vi "JKISM++ List Modules.vi"(8 "Error in":errorcluster caption="Error in (no error)", 9 "Exclude Standalone JKISM(T)":bool=TRUE) -> (0 "Error out":errorcluster, 3 "Module Names":string[](array[string]))   [LabVIEW 2014, in "JKI State Machine++.lvlib"]
doc: "List all JKISM++ Modules alive in system.\n\n<b>Inputs:</b>\n - <b>Exclude Standalone JKISM(T)</b>: 'TRUE' to exclude standalone JKISM module, and 'FALSE' to include them.\n - <b>Error in</b>: Error cluster\n\n<b>Outputs:</b>\n - <b>Module Names</b>: Module Names\n - <b>Error out</b>: Error cluster"
uses:
  JKI State Machine++.lvlib
  _Support/JKISMQ/_JKISMQFGVOPER.ctl
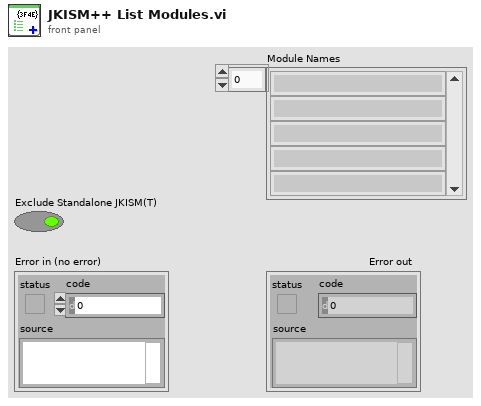
[diagram p1: front panel]
types:
  T1 = typedef "JKI State Machine++.lvlib/_JKISMQFGVOPER.ctl" = enum16{"Get By Name", "List", "Check If Name Exists", "Release", "Module Status"}
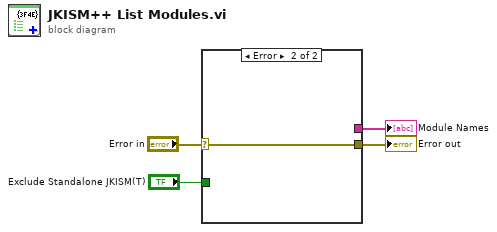
[diagram p0: block diagram]
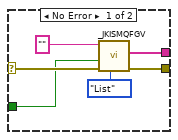
[diagram p2: hidden frame]
diagram:
  n1 = case shown="Error" "Error in" {
    selector: "Error in" -> [w10 w11]
    tunnel: [w9 w11] -> w3
    tunnel: [w6 _] -> w2
    tunnel: "Exclude Standalone JKISM(T)" -> [w5 _]
    frame No Error {
      n2 = call "_JKISMQFGV.vi"("Operation"=_JKISMQFGVOPER."List", "Error in"=w10, "create if not found? (T)"=w5, "Name(\"\" to use uuid) in"="" ("Name(\"\" to use uuid) in")) -> ("Error out"=w9:errorcluster, "Name"=w6:string[])  [unwired: 4 in, 2 out]
    }
    frame Error {
    }
  }
  "Error out" <- w3
  "Module Names" <- w2
